vi "Get End Tag.vi"(8 "error in (no error)":errorcluster, 11 "Element in":refnum<class "Element.lvclass">) -> (0 "error out":errorcluster, 2 "End Tag":string, 3 "Element out":refnum<class "Element.lvclass">)   [LabVIEW 2026, in "VILab.lvlib" / "Element.lvclass"]
uses:
  Element.lvclass
  Data Item/Data Item.lvclass
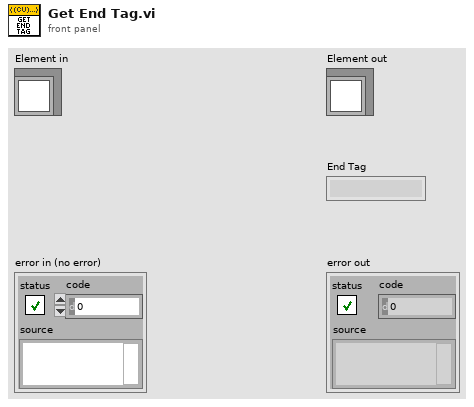
[diagram p1: front panel]
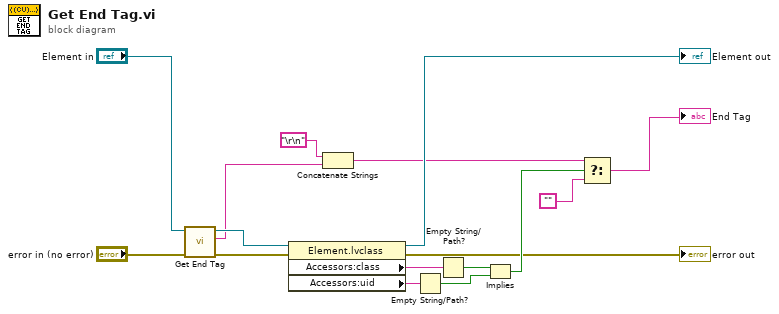
[diagram p0: block diagram]
diagram:
  n1 = call-parent "Get End Tag.vi"("error in (no error)"="error in (no error)", "Data Item in"="Element in") -> ("error out"=w8:errorcluster, "End Tag"=w7:string, "Data Item out"=w9:refnum<class "Element.lvclass">)  [unwired: 7 in]
  n2 = property class="Element.lvclass"(reference=w9, error in=w8) -> (reference out=→"Element out":refnum<class "Element.lvclass">, error out=→"error out":errorcluster, "Accessors:class"=w15:string, "Accessors:uid"=w14:string)
  n3 = Concatenate Strings("\r\n", w7) -> (w3:string)
  n4 = Empty String/Path?(string/path=w14) -> (empty?=w12:bool)
  n5 = Empty String/Path?(string/path=w15) -> (empty?=w13:bool)
  n6 = Implies(1:w12, 2:w13) -> (0:w5:bool)
  n7 = Select(t=w3, s=w5, f="") -> (s? t:f=→"End Tag":string)
